vi "FTW-DevUtil-StaticLinks.vi"(0 "VI Ref":refnum<vi>, 5 "Include Dependencies?":bool, 11 "error in":errorcluster) -> (6 "Files in Project but with no static link here":path[](array[path]), 8 "Files with static link here":path[](array[path]), 15 "error out":errorcluster)   [LabVIEW 2015]
panel:
  # "Inputs"
  # "Outputs"
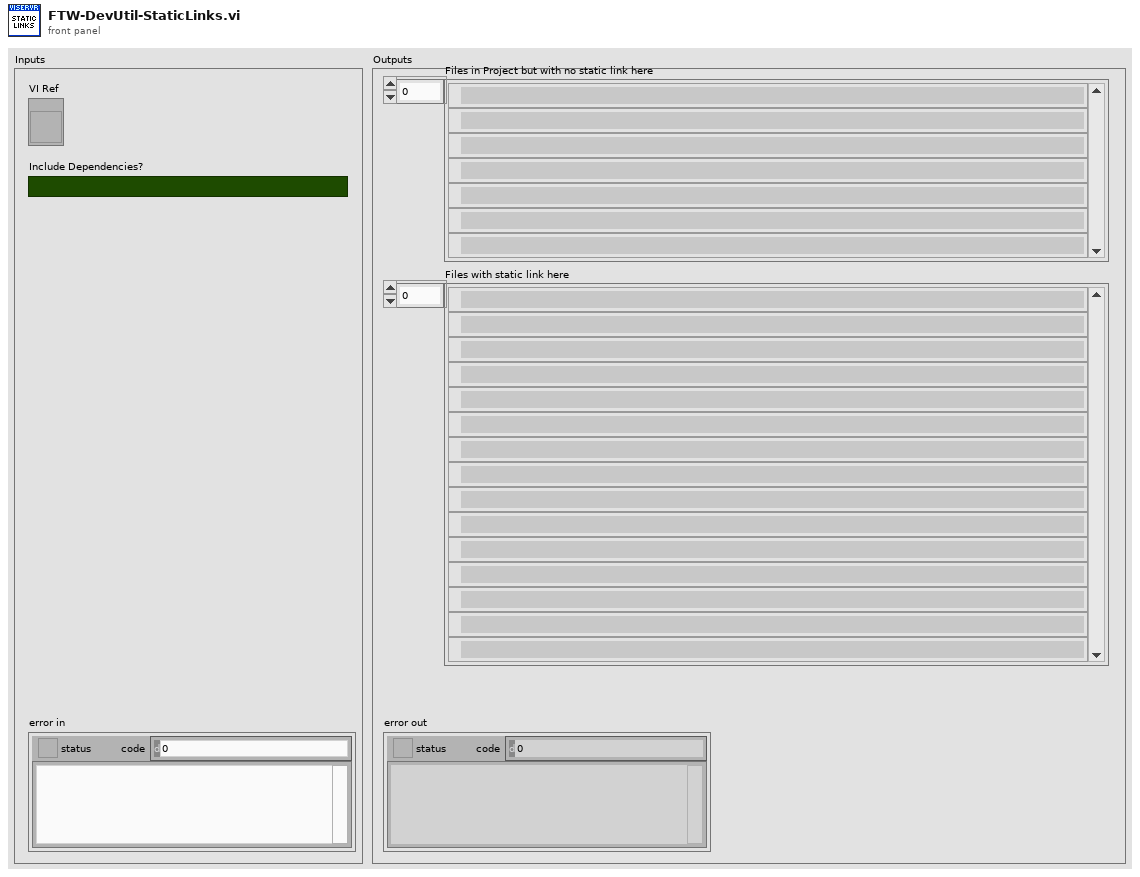
[diagram p1: front panel]
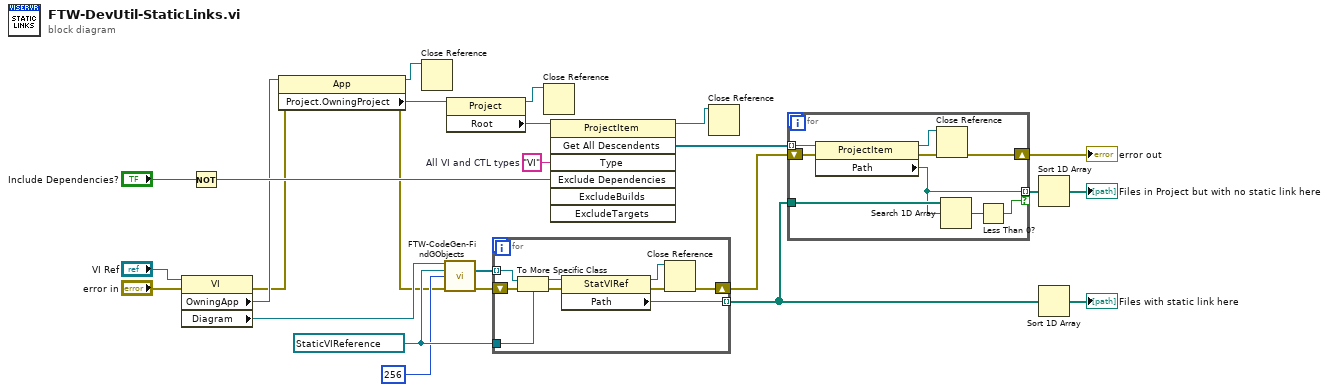
[diagram p0: block diagram]
diagram:
  w19 = "VI"  # All VI and CTL types
  w22 = refnum<vi> refnum ("Block Diagram")
  n1 = property class="VI"(reference="VI Ref", error in="error in") -> (error out=w12:errorcluster, "OwningApp"=w13:refnum<vi>, "Diagram"=w25:refnum<vi>)  [unwired: 1 out]
  n2 = Not(x="Include Dependencies?") -> (.not. x?=w14:bool)
  n3 = property class="App"(reference=w13, error in=w12) -> (reference out=w4:refnum<vi>, error out=w11:errorcluster, "Project.OwningProject"=w21:refnum<vi>)
  n4 = Close Reference(reference=w4) -> ()  [unwired: 1 in, 1 out]
  n5 = call "FTW-CodeGen-FindGObjects.vi"("GObject to Traverse"=w25, "Class Type Reference"=w22, "Maximum Expected Object Count"=256, "error in"=w11) -> ("GObject Instances"=w24:refnum<vi>[], "error out"=w23:errorcluster)  [unwired: 10 in]
  n6 = property class="Project"(reference=w21) -> (reference out=w3:refnum<vi>, "Root"=w20:refnum<vi>)  [unwired: 1 in, 1 out]
  n7 = for {
    tunnel: w24 -> [w33] mode=indexing
    tunnel: w22 -> [w32]
    tunnel: [w29] -> w16 mode=indexing
    shift-right: [w27] -> w2
    shift-left: w23 -> [w34]
    n8 = To More Specific Class(target class=w32, reference=w33, error in=w34) -> (specific class reference=w30:refnum<vi>, error out=w31:errorcluster)
    n9 = property class="StatVIRef"(reference=w30, error in=w31) -> (reference out=w26:refnum<vi>, error out=w28:errorcluster, "Path"=w29:path)
    n10 = Close Reference(reference=w26, error in (no error)=w28) -> (error out=w27:errorcluster)
  }
  n11 = Close Reference(reference=w3) -> ()  [unwired: 1 in, 1 out]
  n12 = invoke class="ProjectItem" method="Get All Descendents"(reference=w20, "Type"=w19, "Exclude Dependencies"=w14) -> (reference out=w5:refnum<vi>, "All Descendents"=w18:refnum<vi>[])  [unwired: 4 in, 5 out]
  n13 = Close Reference(reference=w5) -> ()  [unwired: 1 in, 1 out]
  n14 = for {
    tunnel: w18 -> [w43] mode=indexing
    tunnel: w16 -> [w42]
    tunnel: [w40] -> w17 mode=indexing if=w39
    shift-right: [w35] -> w1
    shift-left: w2 -> [w37]
    n15 = property class="ProjectItem"(reference=w43, error in=w37) -> (reference out=w38:refnum<vi>, error out=w36:errorcluster, "Path"=w40:path)
    n16 = Close Reference(reference=w38, error in (no error)=w36) -> (error out=w35:errorcluster)
    n17 = Search 1D Array(1D array=w42, element=w40) -> (index of element=w41:i32)  [unwired: 1 in]
    n18 = Less Than 0?(x=w41) -> (x < 0?=w39:bool)
  }
  "error out" <- w1
  n19 = Sort 1D Array(array=w17) -> (sorted array=→"Files in Project but with no static link here":path[])
  n20 = Sort 1D Array(array=w16) -> (sorted array=→"Files with static link here":path[])
